vi "ep_Peak Interpolation.vi"(8 "error in (no error)":errorcluster, 10 "magnitude":dbl[](array[numeric]), 11 "frequency [Hz]":dbl[](array[numeric])) -> (0 "error out":errorcluster, 2 "fitted peak magnitude":dbl, 3 "fitted peak frequency":dbl)   [LabVIEW 2014, in "NI_EP_Motor Monitoring.lvlib"]
uses:
  <vilib>/addons/Electrical Power/Motor Monitoring/NI_EP_Motor Monitoring.lvlib
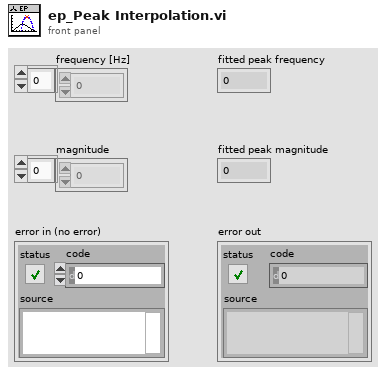
[diagram p1: front panel]
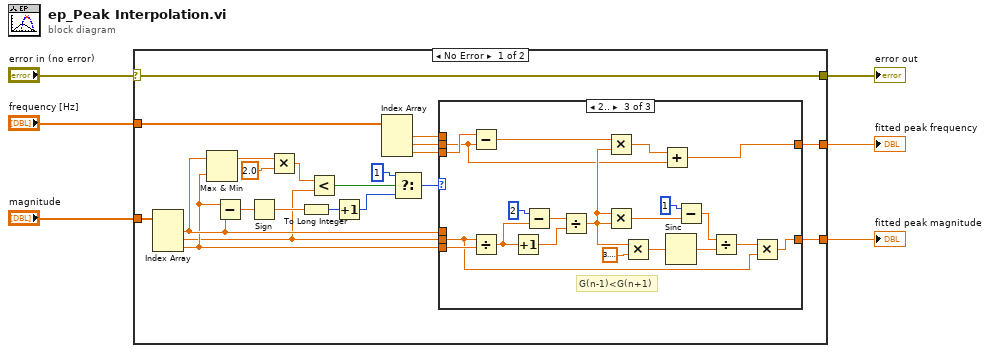
[diagram p0: block diagram]
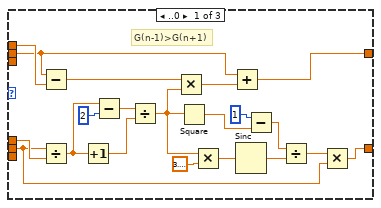
[diagram p2: hidden frame]
diagram:
  n1 = case shown="No Error" "error in (no error)" {
    selector: "error in (no error)" -> [w17 w70]
    tunnel: [w17 w70] -> w5
    tunnel: "frequency [Hz]" -> [w26 _]
    tunnel: "magnitude" -> [w27 _]
    tunnel: [w19 _] -> w2
    tunnel: [w18 _] -> w1
    frame No Error {
      n2 = Index Array(array=w27) -> (element #1=w16:dbl, element #2=w8:dbl, element #3=w15:dbl)  [unwired: 3 in]
      n3 = Max & Min(x=w16, y=w15) -> (max(x,y)=w14:dbl)  [unwired: 1 out]
      n4 = Subtract(x=w15, y=w16) -> (x-y=w23:dbl)
      n5 = Sign(1:w23) -> (0:w25:dbl)
      n6 = Multiply(x=w14, y=2.0) -> (x*y=w9:dbl)
      n7 = To Long Integer(number=w25) -> (32bit integer=w24:i32)
      n8 = Less?(x=w9, y=w8) -> (x < y?=w7:bool)
      n9 = Increment(x=w24) -> (x+1=w11:i32)
      n10 = Index Array(array=w26) -> (element #1=w21:dbl, element #2=w22:dbl, element #3=w20:dbl)  [unwired: 3 in]
      n11 = Select(t=1, s=w7, f=w11) -> (s? t:f=w10:i32)
      n12 = case shown="2.." w10 {
        tunnel: w15 -> [_ _ w60]
        tunnel: w8 -> [w28 w49 w52]
        tunnel: w16 -> [w37 _ _]
        tunnel: [w42 w49 w61] -> w18
        tunnel: w22 -> [w34 w48 w51]
        tunnel: w21 -> [w36 _ _]
        tunnel: w20 -> [_ _ w57]
        tunnel: [w32 w48 w55] -> w19
        frame ..0 {
          # "G(n-1)>G(n+1)"
          n13 = Subtract(x=w34, y=w36) -> (x-y=w35:dbl)
          n14 = Divide(x=w28, y=w37) -> (x/y=w40:dbl)
          n15 = Increment(x=w40) -> (x+1=w46:dbl)
          n16 = Subtract(x=w40, y=2) -> (x-y=w47:dbl)
          n17 = Divide(x=w47, y=w46) -> (x/y=w30:dbl)
          n18 = Multiply(x=w35, y=w30) -> (x*y=w33:dbl)
          n19 = Square(x=w30) -> (x^2=w31:dbl)
          n20 = Multiply(x=w30, y=3.141592653589793) -> (x*y=w41:dbl)
          n21 = Add(x=w34, y=w33) -> (x+y=w32:dbl)
          n22 = Sinc(1:w41) -> (0:w38:dbl)
          n23 = Subtract(x=1, y=w31) -> (x-y=w43:dbl)
          n24 = Divide(x=w43, y=w38) -> (x/y=w29:dbl)
          n25 = Multiply(x=w29, y=w28) -> (x*y=w42:dbl)
        }
        frame 1 {
          # "G(n-1)=G(n+1)\nor\nG(n)>2*max(G(n-1),G(n+1))"
        }
        frame 2.. {
          # "G(n-1)<G(n+1)"
          n26 = Subtract(x=w57, y=w51) -> (x-y=w56:dbl)
          n27 = Divide(x=w52, y=w60) -> (x/y=w68:dbl)
          n28 = Increment(x=w68) -> (x+1=w66:dbl)
          n29 = Subtract(x=2, y=w68) -> (x-y=w67:dbl)
          n30 = Divide(x=w67, y=w66) -> (x/y=w54:dbl)
          n31 = Multiply(x=w56, y=w54) -> (x*y=w50:dbl)
          n32 = Multiply(x=w54, y=w54) -> (x*y=w63:dbl)
          n33 = Multiply(x=w54, y=3.141592653589793) -> (x*y=w58:dbl)
          n34 = Add(x=w50, y=w51) -> (x+y=w55:dbl)
          n35 = Sinc(1:w58) -> (0:w59:dbl)
          n36 = Subtract(x=1, y=w63) -> (x-y=w62:dbl)
          n37 = Divide(x=w62, y=w59) -> (x/y=w53:dbl)
          n38 = Multiply(x=w53, y=w52) -> (x*y=w61:dbl)
        }
      }
    }
    frame Error {
    }
  }
  "error out" <- w5
  "fitted peak frequency" <- w2
  "fitted peak magnitude" <- w1
